vi "SPVM-to-PrintInfo.vi"() -> ()   [LabVIEW 2020]
uses:
  <vilib>/Math Plots/3D Math Plots/3D Scatter/3D Scatter XCtrl/3D Scatter.xctl
  <vilib>/Utility/error.llb/Error Cluster From Error Code.vi
  <vilib>/Math Plots/3D Math Plots/3D Scatter/3D Scatter Datatype/Public/Plot Helper (Vector).vi
  <vilib>/ErrorRing/Error Ring.xnode
  <vilib>/Math Plots/3D Math Plots/3D Plot/3D Plot Datatype/3D Plot Datatype.lvclass
  <vilib>/Math Plots/3D Math Plots/3D Scatter/3D Scatter Datatype/3D Scatter Datatype.lvclass
panel:
  in  "file (use dialog)":path=path "C:/Users/Lexa/DevProjects/Prometheus/Scalable packed voxel mapping/test.spvm"
  in  "Boolean":bool
  out "Voxel qty":i32
  out "m3 before\noverflow":ext
  out "VoxelData":u8[](array[numeric])
  out "Metadata":T1
  out "Next Vector #":u8
  out "Current vector":i8[](array[numeric])
  out "Current position":i8[](array[numeric])
  out "Ring position":u64
  in  "Slow?":bool=TRUE
  in  "Rings to render ( mock )":i32=24
  out "3D Scatter":refnum<class "3D Plot Datatype.lvclass">[](xcontrol)
  out "Index":u64 format="%^.3e"
  out "output array":T2(array[cluster]) {"d" format="%02x"}
  out "Voxels ( Cartesian )":dbl[][](array[numeric])
  out "Values at index":i64[](array[numeric]) caption="Values at index\n( Vox index, Ring index, nth ring vox, 0-nth ring £ )"
  out "Current ring":i64
  out "Ring size":i64
  out "Boolean 2":bool
  out "message":string=" INSTRUCTIONS:\r\rNormal Use:  When using subVIs that incorporate the error in/error out (or error I/O) structure, place this handler where you want to inform the user of an error, typically at the end of the I/O data path, as the last action of the program.  If the error in error? is ERROR, the handler creates a message describing the error and its source.  If the type of dialog = 1 (default), the message is displayed to the user, who can only acknowedge it.  If the type = 2, the user can acknowledge the message or abort execution; aborting a program with active I/O is not recommended.  If the type = 0, no message is displayed; this is used to process the error programmatically, and the error out cluster elements are wired to individual terminals for that reason.  \r\rOther Use:\n\r\nlocal testing.  To test the error code of a subVI or function that does not have the error I/O structure, you can wire its error code and a source string to the local error code and error source inputs.  If error in error? indicates no error and error code is not equal to 0, the local code and source are substituted for the error in values, and error? is set TRUE (ERROR)."
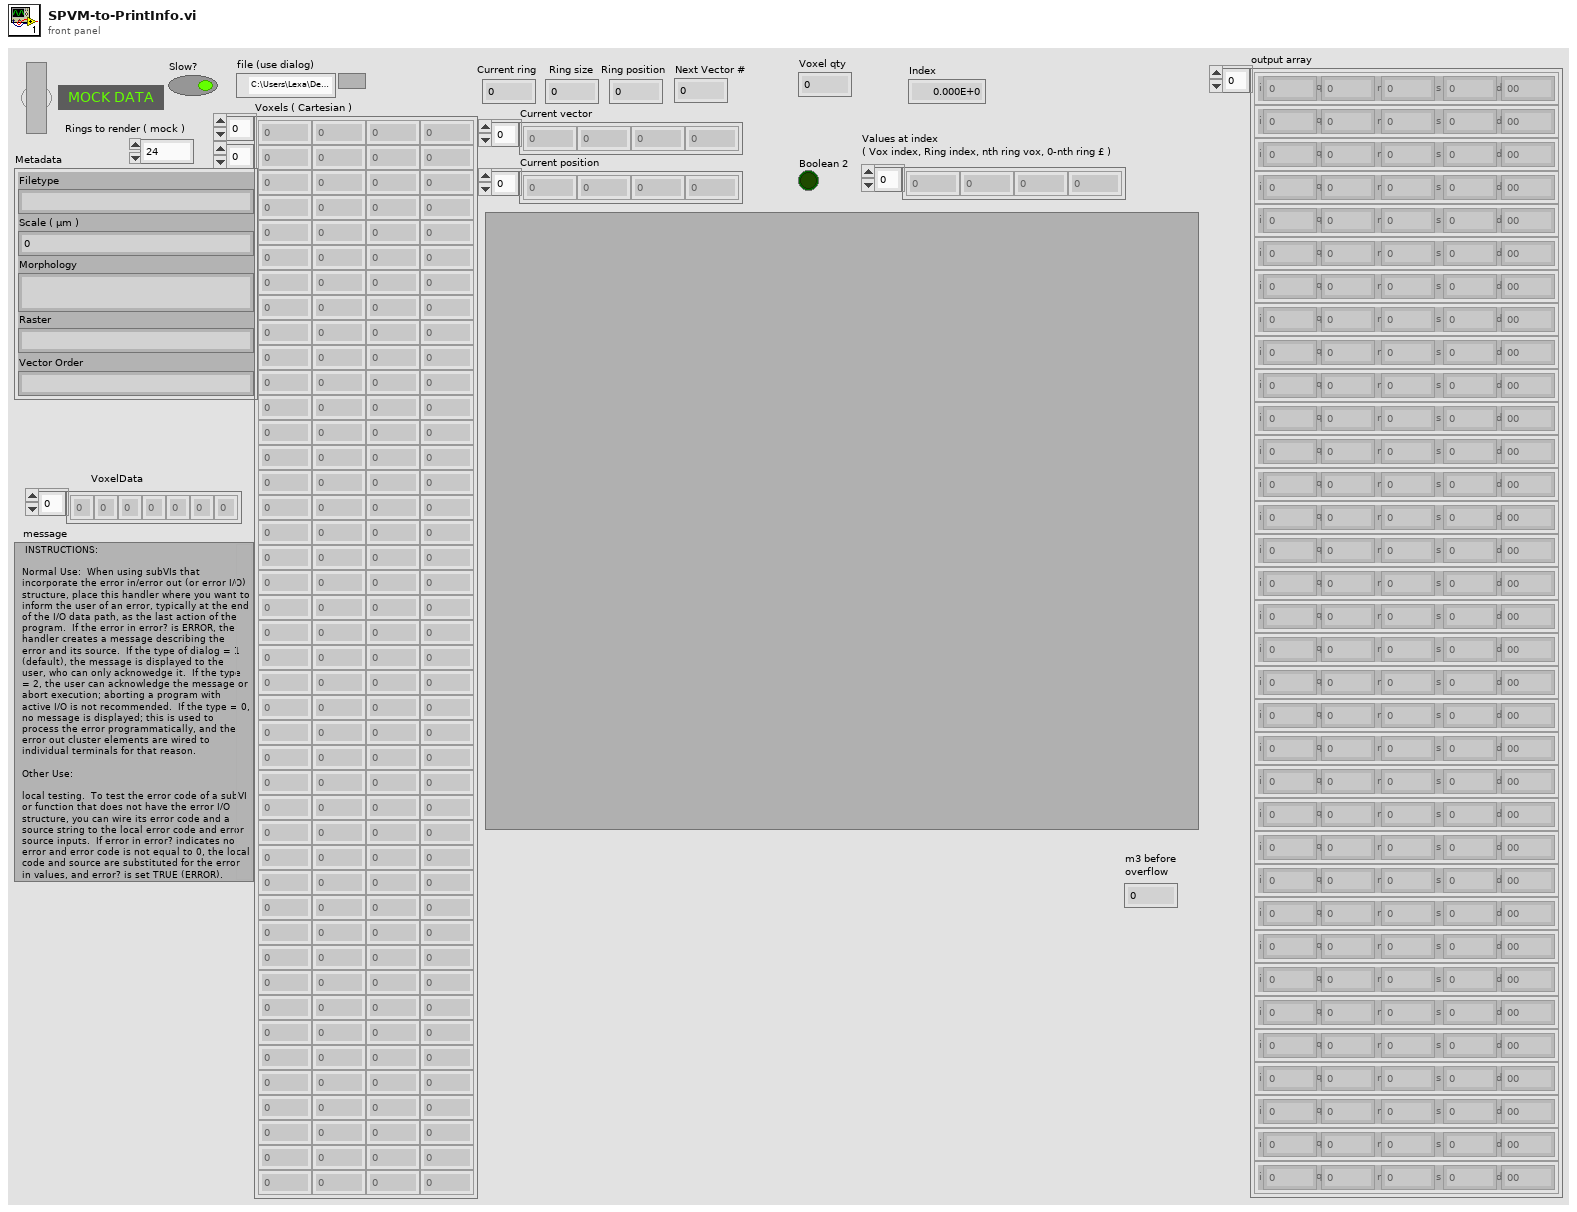
[diagram p1: front panel]
types:
  T1 = cluster{"Filetype":string, "Scale ( µm )":ext, "Morphology":string, "Raster":string, "Vector Order":string}
  T2 = cluster{"i":u64, "q":i64, "r":i64, "s":i64, "d":u8}[]
  T3 = cluster{"Filetype":string, "Scale ( µm )":ext, "Morphology":string, "Raster":string, "VectorOrder":string}
  T4 = cluster{"i":u64, "q":i64, "r":i64, "s":i64, "d":u8}
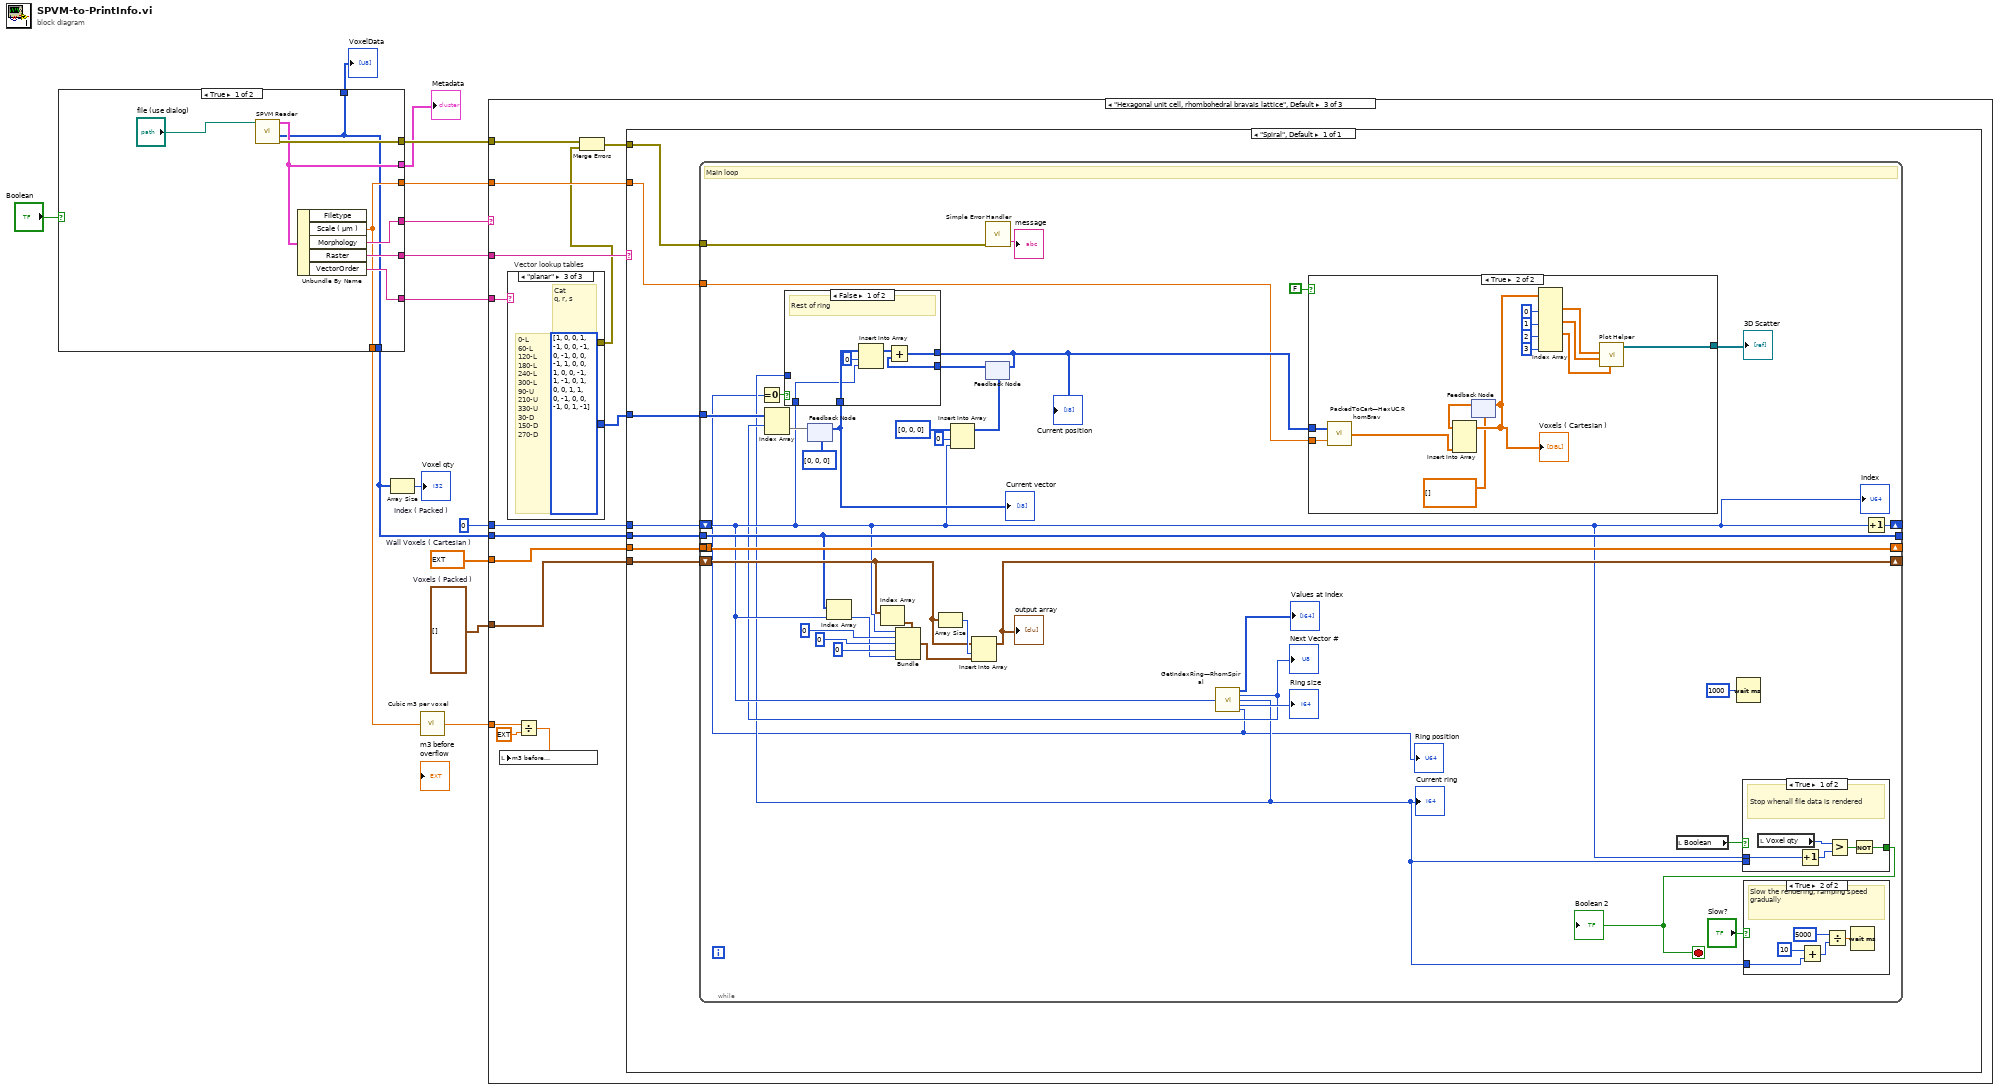
[diagram p0: block diagram]
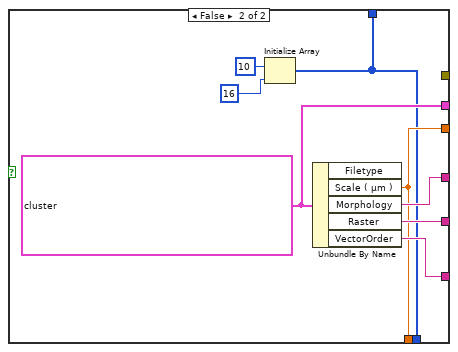
[diagram p2: hidden frame]
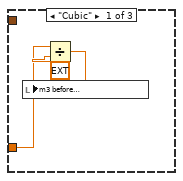
[diagram p3: hidden frame]
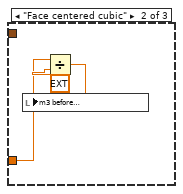
[diagram p4: hidden frame]
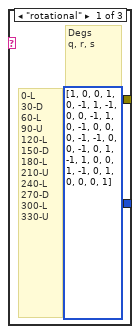
[diagram p5: hidden frame]
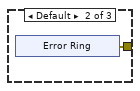
[diagram p6: hidden frame]
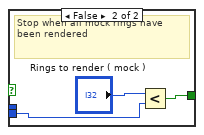
[diagram p8: hidden frame]
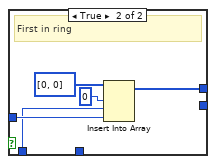
[diagram p10: hidden frame]
diagram:
  w4 = T2 []  # Voxels ( Packed )
  w10 = ext[] [0.0, 0.0, 0.0]  # Wall Voxels ( Cartesian )
  w13 = u64 0  # Index ( Packed )
  n1 = case shown="True" "Boolean" {
    tunnel: [w22 w31] -> w15
    tunnel: [w21 w30] -> w14
    tunnel: [w20 _] -> w12
    tunnel: [w19 w29] -> w11
    tunnel: [w17 w28] -> w9
    tunnel: [w18 w27] -> w6
    tunnel: [w17 w28] -> w5
    tunnel: [w16 w24] -> w3
    tunnel: [w16 w24] -> w2
    frame True {
      n2 = call "SPVM Reader.vi"("file (use dialog)"="file (use dialog)") -> ("error out"=w20:errorcluster, "VoxelData"=w16:u8[], "Metadata"=w18:T3)  [unwired: 6 in, 2 out]
      n3 = Unbundle By Name(w18) -> ("Scale ( µm )"=w17:ext, "Morphology"=w22:string, "Raster"=w21:string, "VectorOrder"=w19:string)  [unwired: 1 out]
    }
    frame False {
      w27 = T3 {"Filetype"="MOCKDATA", "Scale ( µm )"=50.0, "Morphology"="hexagonal unit cell, rhombohedral bravais lattice", "Raster"="spiral", "VectorOrder"="planar"} ("input cluster")
      n4 = Initialize Array(u8 10 ("element"), 16 ("dimension size")) -> (w24:u8[])
      n5 = Unbundle By Name(w27) -> ("Scale ( µm )"=w28:ext, "Morphology"=w31:string, "Raster"=w30:string, "VectorOrder"=w29:string)  [unwired: 1 out]
    }
  }
  "Metadata" <- w6
  "VoxelData" <- w2
  n6 = Array Size(array=w3) -> (size(s)=→"Voxel qty":i32)
  n7 = call "Cubic m3 per voxel.vi"("Scale ( µm )"=w5) -> ("Numeric"=w8:ext)  [unwired: 7 in, 1 out]
  n8 = case shown="\"Hexagonal unit cell, rhombohedral bravais lattice\", Default" w15 {
    tunnel: w14 -> [_ _ w51]
    tunnel: w9 -> [_ _ w50]
    tunnel: w12 -> [_ _ w46]
    tunnel: w13 -> [_ _ w48]
    tunnel: w11 -> [_ _ w47]
    tunnel: w10 -> [_ _ w40]
    tunnel: w8 -> [w32 w35 w43]
    tunnel: w3 -> [_ _ w39]
    tunnel: w4 -> [_ _ w38]
    frame "Cubic" {
      n9 = Divide(x=w32, y=ext 1.0) -> (x/y=w33:ext)
      n10 = local write "m3 before\noverflow"(w33) -> ()
    }
    frame "Face centered cubic" {
      n11 = Divide(x=w35, y=ext 4.0) -> (x/y=w36:ext)
      n12 = local write "m3 before\noverflow"(w36) -> ()
    }
    frame "Hexagonal unit cell, rhombohedral bravais lattice", Default {
      n13 = case "Vector lookup tables" shown="\"planar\"" w47 {
        tunnel: [i8[][] [[1, 0, 0], [1, 0, -1], [1, -1, 0], [0, -1, 1], [0, -1, 0], [0, 0, -1], [-1, 0, 0], [-1, 0, 1], [-1, 1, 0], [0, 1, -1], [0, 1, 0], [0, 0, 1]] _ i8[][] [[1, 0, 0], [1, -1, 0], [0, -1, 0], [-1, 0, 0], [-1, 1, 0], [0, 1, 0], [0, -1, 1], [-1, 0, 1], [0, 0, 1], [1, 0, -1], [0, 0, -1], [0, 1, -1]]] -> w49
        tunnel: [_ w53 _] -> w44
        frame "rotational" {
          # "0-L\n30-D\n60-L\n90-U\n120-L\n150-D\n180-L\n210-U\n240-L\n270-D\n300-L\n330-U"
          # "Degs \nq, r, s"
        }
        frame Default {
          n14 = xnode "Error Ring"() -> ("error out"=w53:errorcluster)
        }
        frame "planar" {
          # "0-L\n60-L\n120-L\n180-L\n240-L\n300-L\n90-U\n210-U\n330-U\n30-D\n150-D\n270-D"
          # "Cat \nq, r, s"
        }
      }
      n15 = Divide(x=w43, y=ext 4.0) -> (x/y=w41:ext)
      n16 = local write "m3 before\noverflow"(w41) -> ()
      n17 = Merge Errors(w46, w44) -> (w45:errorcluster)
      n18 = case shown="\"Spiral\", Default" w51 {
        tunnel: w50 -> [w62]
        tunnel: w49 -> [w65]
        tunnel: w45 -> [w64]
        tunnel: w48 -> [w63]
        tunnel: w40 -> [w61]
        tunnel: w39 -> [w60]
        tunnel: w38 -> [w59]
        frame "Spiral", Default {
          n19 = while {
            tunnel: w65 -> [w102]
            tunnel: w62 -> [w90]
            shift-right: [w88] -> _
            shift-left: w63 -> [w71]
            tunnel: w61 -> [w87]
            shift-right: [w87] -> _
            shift-left: _ -> [_]
            tunnel: w60 -> [w78]
            tunnel: [w78] -> _
            shift-right: [w80] -> _
            shift-left: w59 -> [w85]
            tunnel: w64 -> [w72]
            stop <- w74 stop-if-true
            # "Main loop"
            n20 = feedback #1(i8[] [0, 0, 0] ("x")) -> (w99:i8[])
            "Current vector" <- w99
            n21 = Index Array(array=w78, index=w71) -> (element=w77:u8)
            n22 = Index Array(array=w85) -> (element=w84:T4)  [unwired: 1 in]
            n23 = Bundle(cluster=w84, "i"=w71, "q"=i64 0, "r"=i64 0, "s"=i64 0, "d"=w77) -> (w83:T4)
            n24 = Array Size(array=w85) -> (size(s)=w86:i32)
            n25 = Insert Into Array(array=i8[] [0, 0, 0] ("x"), index=0, new element=w71) -> (w94:i8[])
            n26 = Insert Into Array(array=w85, index=w86, new element=w83) -> (w80:T2)
            "output array" <- w80
            n27 = feedback #2(w94) -> (w98:i8[])
            n28 = call <vilib>:"Simple Error Handler.vi"("error in (no error)"=w72) -> ("message"=→"message":string)  [unwired: 4 in, 4 out]
            n29 = call "GetIndexRing—RhomSpiral.vi"("Index"=w71) -> ("Values at index"=→"Values at index":i64[], "Next vector #"=w68:u8, "Current ring"=w67:i64, "Ring size"=→"Ring size":i64, "Ring position"=w66:u64)  [unwired: 10 in]
            "Next Vector #" <- w68
            "Ring position" <- w66
            "Current ring" <- w67
            n30 = Equal To 0?(x=w66) -> (x = 0?=w100:bool)
            n31 = Index Array(array=w102, index (row)=w68) -> (element=w96:i8[])  [unwired: 1 in]
            n32 = case shown="False" w100 {
              tunnel: w67 -> [_ w137]
              tunnel: w99 -> [w133 _]
              tunnel: [w135 w138] -> w91
              tunnel: w98 -> [w134 _]
              tunnel: w71 -> [w130 w136]
              frame False {
                # "Rest of ring"
                n33 = Insert Into Array(array=w133, index=0, new element=w130) -> (w132:i8[])
                n34 = Add(x=w132, y=w134) -> (x+y=w135:i8[])
              }
              frame True {
                # "First in ring"
                n35 = Insert Into Array(array=i8[] [0, 0] ("x"), index=0, new element #1=w136, new element #2=w137) -> (w138:i8[])
              }
            }
            "Current position" <- w91
            n36 = feedback-in #1(w96) -> ()
            n37 = feedback-in #2(w91) -> ()
            n38 = case shown="True" FALSE {
              tunnel: w91 -> [_ w115]
              tunnel: w90 -> [_ w114]
              tunnel: [_ w113] -> w89
              frame False {
              }
              frame True {
                n39 = call "PackedToCart—HexUC,RhomBrav.vi"("Scale mult. ( um )"=w114, "Packed coordinates ( qword 1D array )"=w115) -> ("Cartesian coordinates ( double 1D array )"=w103:dbl[])
                n40 = feedback #3(dbl[][] []) -> (w116:dbl[][])
                n41 = Insert Into Array(array=w116, new element=w103) -> (w108:dbl[][])  [unwired: 2 in]
                "Voxels ( Cartesian )" <- w108
                n42 = feedback-in #3(w108) -> ()
                n43 = Index Array(array=w108, index (col) #1=0 ("disabled index (col)"), index (col) #2=1 ("index (col)"), index (col) #3=2 ("index (col)"), index (col) #4=3 ("index (col)")) -> (element #1=w107:dbl[], element #2=w106:dbl[], element #3=w105:dbl[])  [unwired: 4 in, 1 out]
                n44 = call-poly <vilib>:"Plot Helper.vi"("z vector"=w105, "y vector"=w106, "x vector"=w107) -> ("3D Plot lvclass Array out"=w113:refnum<class "3D Plot Datatype.lvclass">[])  [unwired: 3 in, 5 out]
              }
            }
            "3D Scatter" <- w89
            n45 = local read "Boolean"() -> (w92:bool)
            n46 = Wait (ms)(milliseconds to wait=u32 1000) -> ()  [unwired: 1 out]
            n47 = case shown="True" w92 {
              tunnel: [w119 w123] -> w74
              tunnel: w71 -> [w118 _]
              tunnel: w67 -> [_ w122]
              frame True {
                # "Stop whenall file data is rendered"
                n48 = local read "Voxel qty"() -> (w121:i32)
                n49 = Increment(x=w118) -> (x+1=w117:u64)
                n50 = Greater?(x=w121, y=w117) -> (0:w120:bool)
                n51 = Not(x=w120) -> (.not. x?=w119:bool)
              }
              frame False {
                # "Stop when all mock rings have been rendered"
                n52 = Less?(x="Rings to render ( mock )", y=w122) -> (x < y?=w123:bool)
              }
            }
            "Boolean 2" <- w74
            n53 = case shown="True" "Slow?" {
              tunnel: w67 -> [_ w128]
              frame False {
                # "Render as fast as system allows"
              }
              frame True {
                # "Slow the rendering, ramping speed gradually"
                n54 = Add(x=10, y=w128) -> (x+y=w126:i64)
                n55 = Divide(x=5000, y=w126) -> (x/y=w125:dbl)
                n56 = Wait (ms)(milliseconds to wait=w125) -> ()  [unwired: 1 out]
              }
            }
            n57 = Increment(x=w71) -> (x+1=w88:u64)
            "Index" <- w71
          }
        }
      }
    }
  }
